vi "Camera_Config_Global_Attributes.vi"(7 "Camera":T1, 8 "error in (no error)":errorcluster, 10 "Refnum in":T3, 11 "input cluster":T2={"Pinch-valve"="", "XLP 6000 Pump"="", "Camera1"="", "Camera2"="", "Img_Capt"=FALSE, "Actuator"=FALSE, "Pump"=FALSE, "Cam 1"=FALSE, "Cam 2"=FALSE, "Empty_Refill"=FALSE, "Crop"=FALSE, "Light intensity"=0, "Exposure Time"=0.0, "Sample Name"="", "Operator"="", "Calibration 1"=path "", "Calibration 2"=path "", "Framerate"=0, "Timeout Sample"=0, "Collection date"="", "Sample size threshold"=0, "Empty start"=0, "Command"="", "Station"="", "Species Name"="", "Other Notes"="", "Aperture"=enum."Item 0", "Image Process Queue Size"=0, "Image Save Queue Size"=0, "Overload threshold"=0, "Max Framerate"=0, "Rectangle 1"={"Left"=0, "Top"=0, "Right"=0, "Bottom"=0, "Rotation"=0.0}, "Rectangle 2"={"Left"=0, "Top"=0, "Right"=0, "Bottom"=0, "Rotation"=0.0}, "Detection Region %"=200.0, "Detect 1"=path "", "Detect 2"=path "", "Max large object threshold"=500, "Open(T)/Close(F)"=FALSE, "Img_Capt Begin"=FALSE, "Dispense Speed"=0, "Flush Size"=0, "Location"="", "Latitude"="", "Longitude"="", "Determiner"="", "Sex"="", "Camera1_Img"=refnum, "Camera2_Img"=refnum, "Img1_Orig_Disp"=refnum, "Img2_Orig_Disp"=refnum, "Img1_Orig_RGB"=refnum, "Img2_Orig_RGB"=refnum, "Blue_Plane_Extract"=refnum, "Subtracted_Plane"=refnum, "Img1_Binary"=refnum, "Img2_Binary"=refnum, "Crop_Mask"=refnum, "Img1_Save"=refnum, "Img2_Save"=refnum, "Img1_Cali_Full"=refnum, "Img2_Cali_Full"=refnum, "Img1_Cali_Detect"=refnum, "Img2_Cali_Detect"=refnum, "Cam 1 queue"=refnum, "Cam 2 queue"=refnum, "Cam 1 - save queue"=refnum, "Cam 2 - save queue"=refnum, "Overlay_Ring"=0, "SystemVersion"=0, "System Serial"="", "Legacy Cam Attributes"=FALSE, "Camera Orientation 1"="", "Camera Orientation 2"="", "Pixel to mm 1"=0.0, "Pixel to mm 2"=0.0, "CAM1 Model"=enum."a2A5328-15ucBAS", "CAM2 Model"=enum."a2A5328-15ucBAS", "Flush Insect"=FALSE, "Pump Size"=FALSE, "Barcode"="", "Phase3"=FALSE, "Mega F3"="", "Container nr."=0.0, "Flush Error"=TRUE, "Start System"=FALSE, "Size Interval"=0.0, "Mun. of containers"=0.0, "Sorting sys."=FALSE, "Initial size"=0.0} {"SystemVersion" items=["Standard", "XL"]; "Overlay_Ring" items=["Session Data", "Extended Setup", "Buffer", "Camera", "Dispenser", "Stats", "Connections"]; "Flush Size" min=1; "Dispense Speed" min=1; "Rectangle 2"."Rotation" format="%.2f"; "Rectangle 2"."Left" scale=0.0..1024.0; "Rectangle 2"."Right" scale=0.0..1024.0; "Rectangle 1"."Rotation" format="%.2f"; "Rectangle 1"."Left" scale=0.0..1024.0; "Rectangle 1"."Right" scale=0.0..1024.0; "Max Framerate" min=1; "Overload threshold" min=1; "Image Save Queue Size" min=1; "Image Process Queue Size" min=1; "Empty start" min=1; "Sample size threshold" min=1; "Framerate" min=1; "Light intensity" scale=0.0..100.0}) -> (0 "error out":errorcluster, 2 "Refnum out":T3, 3 "input cluster out":T2={"Pinch-valve"="", "XLP 6000 Pump"="", "Camera1"="", "Camera2"="", "Img_Capt"=FALSE, "Actuator"=FALSE, "Pump"=FALSE, "Cam 1"=FALSE, "Cam 2"=FALSE, "Empty_Refill"=FALSE, "Crop"=FALSE, "Light intensity"=0, "Exposure Time"=0.0, "Sample Name"="", "Operator"="", "Calibration 1"=path "", "Calibration 2"=path "", "Framerate"=0, "Timeout Sample"=0, "Collection date"="", "Sample size threshold"=0, "Empty start"=0, "Command"="", "Station"="", "Species Name"="", "Other Notes"="", "Aperture"=enum."Item 0", "Image Process Queue Size"=0, "Image Save Queue Size"=0, "Overload threshold"=0, "Max Framerate"=0, "Rectangle 1"={"Left"=0, "Top"=0, "Right"=0, "Bottom"=0, "Rotation"=0.0}, "Rectangle 2"={"Left"=0, "Top"=0, "Right"=0, "Bottom"=0, "Rotation"=0.0}, "Detection Region %"=200.0, "Detect 1"=path "", "Detect 2"=path "", "Max large object threshold"=500, "Open(T)/Close(F)"=FALSE, "Img_Capt Begin"=FALSE, "Dispense Speed"=0, "Flush Size"=0, "Location"="", "Latitude"="", "Longitude"="", "Determiner"="", "Sex"="", "Camera1_Img"=refnum, "Camera2_Img"=refnum, "Img1_Orig_Disp"=refnum, "Img2_Orig_Disp"=refnum, "Img1_Orig_RGB"=refnum, "Img2_Orig_RGB"=refnum, "Blue_Plane_Extract"=refnum, "Subtracted_Plane"=refnum, "Img1_Binary"=refnum, "Img2_Binary"=refnum, "Crop_Mask"=refnum, "Img1_Save"=refnum, "Img2_Save"=refnum, "Img1_Cali_Full"=refnum, "Img2_Cali_Full"=refnum, "Img1_Cali_Detect"=refnum, "Img2_Cali_Detect"=refnum, "Cam 1 queue"=refnum, "Cam 2 queue"=refnum, "Cam 1 - save queue"=refnum, "Cam 2 - save queue"=refnum, "Overlay_Ring"=0, "SystemVersion"=0, "System Serial"="", "Legacy Cam Attributes"=FALSE, "Camera Orientation 1"="", "Camera Orientation 2"="", "Pixel to mm 1"=0.0, "Pixel to mm 2"=0.0, "CAM1 Model"=enum."a2A5328-15ucBAS", "CAM2 Model"=enum."a2A5328-15ucBAS", "Flush Insect"=FALSE, "Pump Size"=FALSE, "Barcode"="", "Phase3"=FALSE, "Mega F3"="", "Container nr."=0.0, "Flush Error"=TRUE, "Start System"=FALSE, "Size Interval"=0.0, "Mun. of containers"=0.0, "Sorting sys."=FALSE, "Initial size"=0.0} {"SystemVersion" items=["Standard", "XL"]; "Overlay_Ring" items=["Session Data", "Extended Setup", "Buffer", "Camera", "Dispenser", "Stats", "Connections"]; "Flush Size" min=1; "Dispense Speed" min=1; "Rectangle 2"."Rotation" format="%.2f"; "Rectangle 2"."Left" scale=0.0..1024.0; "Rectangle 2"."Right" scale=0.0..1024.0; "Rectangle 1"."Rotation" format="%.2f"; "Rectangle 1"."Left" scale=0.0..1024.0; "Rectangle 1"."Right" scale=0.0..1024.0; "Max Framerate" min=1; "Overload threshold" min=1; "Image Save Queue Size" min=1; "Image Process Queue Size" min=1; "Empty start" min=1; "Sample size threshold" min=1; "Framerate" min=1; "Light intensity" scale=0.0..100.0})   [LabVIEW 2024]
uses:
  controls/Data.ctl
  <vilib>/userDefined/High Color/IMAQdx.ctl
  <vilib>/vision/Image Controls.llb/IMAQ Image.ctl
  Camera_ID.ctl
  <resource>/objmgr/imaqdx.rc
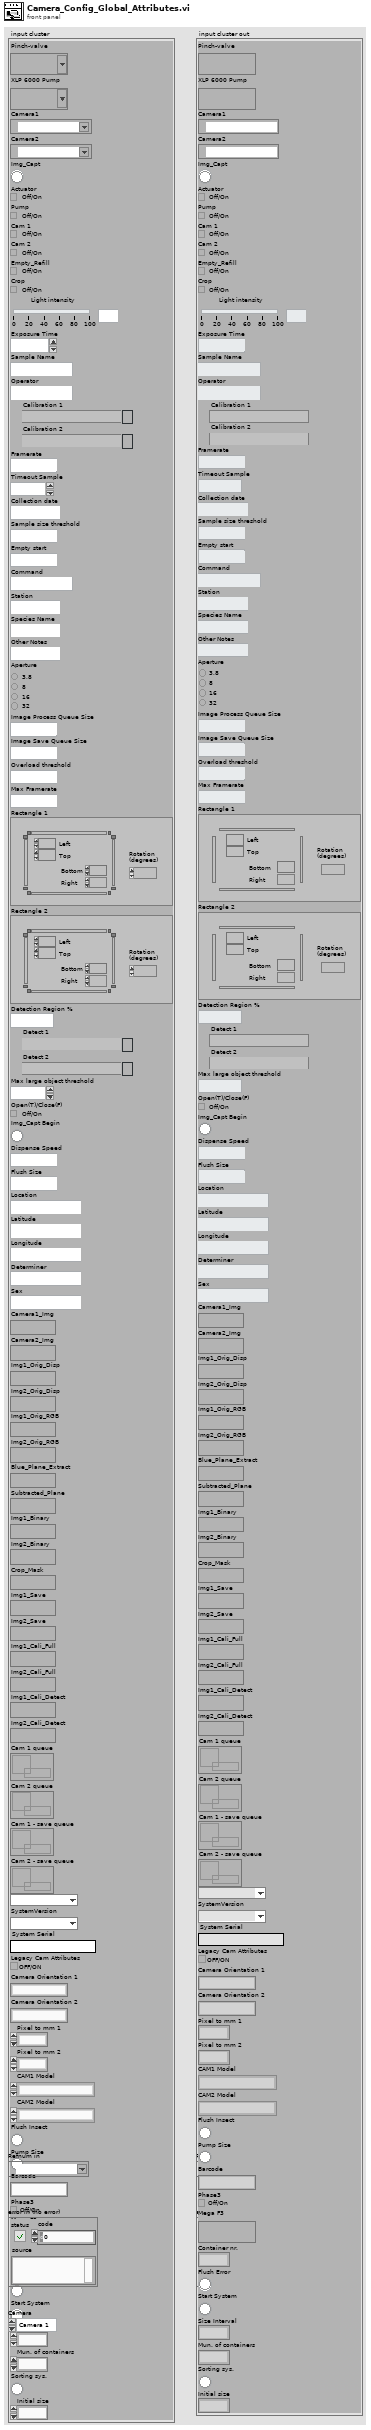
[diagram p1: front panel]
types:
  T1 = typedef "Camera_ID.ctl" = enum16{"Camera 1", "Camera 2"}
  T2 = typedef "Data.ctl" = cluster{"Pinch-valve":refnum<visa-resource-name>, "XLP 6000 Pump":refnum<visa-resource-name>, "Camera1":T3, "Camera2":T3, "Img_Capt":bool, "Actuator":bool, "Pump":bool, "Cam 1":bool, "Cam 2":bool, "Empty_Refill":bool, "Crop":bool, "Light intensity":i32, "Exposure Time":dbl, "Sample Name":string, "Operator":string, "Calibration 1":path, "Calibration 2":path, "Framerate":i32, "Timeout Sample":i32, "Collection date":string, "Sample size threshold":i32, "Empty start":u32, "Command":string, "Station":string, "Species Name":string, "Other Notes":string, "Aperture":enum32{"Item 0", "Item 1", "Item 2", "Item 3"}, "Image Process Queue Size":i32, "Image Save Queue Size":i32, "Overload threshold":i32, "Max Framerate":i32, "Rectangle 1":T4, "Rectangle 2":T4, "Detection Region %":dbl, "Detect 1":path, "Detect 2":path, "Max large object threshold":i32, "Open(T)/Close(F)":bool, "Img_Capt Begin":bool, "Dispense Speed":i32, "Flush Size":i32, "Location":string, "Latitude":string, "Longitude":string, "Determiner":string, "Sex":string, "Camera1_Img":T5, "Camera2_Img":T5, "Img1_Orig_Disp":T5, "Img2_Orig_Disp":T5, "Img1_Orig_RGB":T5, "Img2_Orig_RGB":T5, "Blue_Plane_Extract":T5, "Subtracted_Plane":T5, "Img1_Binary":T5, "Img2_Binary":T5, "Crop_Mask":T5, "Img1_Save":T5, "Img2_Save":T5, "Img1_Cali_Full":T5, "Img2_Cali_Full":T5, "Img1_Cali_Detect":T5, "Img2_Cali_Detect":T5, "Cam 1 queue":refnum<queue>, "Cam 2 queue":refnum<queue>, "Cam 1 - save queue":refnum<queue>, "Cam 2 - save queue":refnum<queue>, "Overlay_Ring":u16, "SystemVersion":u16, "System Serial":string, "Legacy Cam Attributes":bool, "Camera Orientation 1":string, "Camera Orientation 2":string, "Pixel to mm 1":dbl, "Pixel to mm 2":dbl, "CAM1 Model":enum16{"a2A5328-15ucBAS", "acA1920-155uc"}, "CAM2 Model":enum16{"a2A5328-15ucBAS", "acA1920-155uc"}, "Flush Insect":bool, "Pump Size":bool, "Barcode":string, "Phase3":bool, "Mega F3":refnum<visa-resource-name>, "Container nr.":dbl, "Flush Error":bool, "Start System":bool, "Size Interval":dbl, "Mun. of containers":dbl, "Sorting sys.":bool, "Initial size":dbl}
  T3 = typedef "IMAQdx.ctl" = refnum<k21>
  T4 = typedef "IMAQ Rectangle" = cluster{"Left":i32, "Top":i32, "Right":i32, "Bottom":i32, "Rotation":dbl}
  T5 = typedef "IMAQ Image.ctl" = refnum<image>
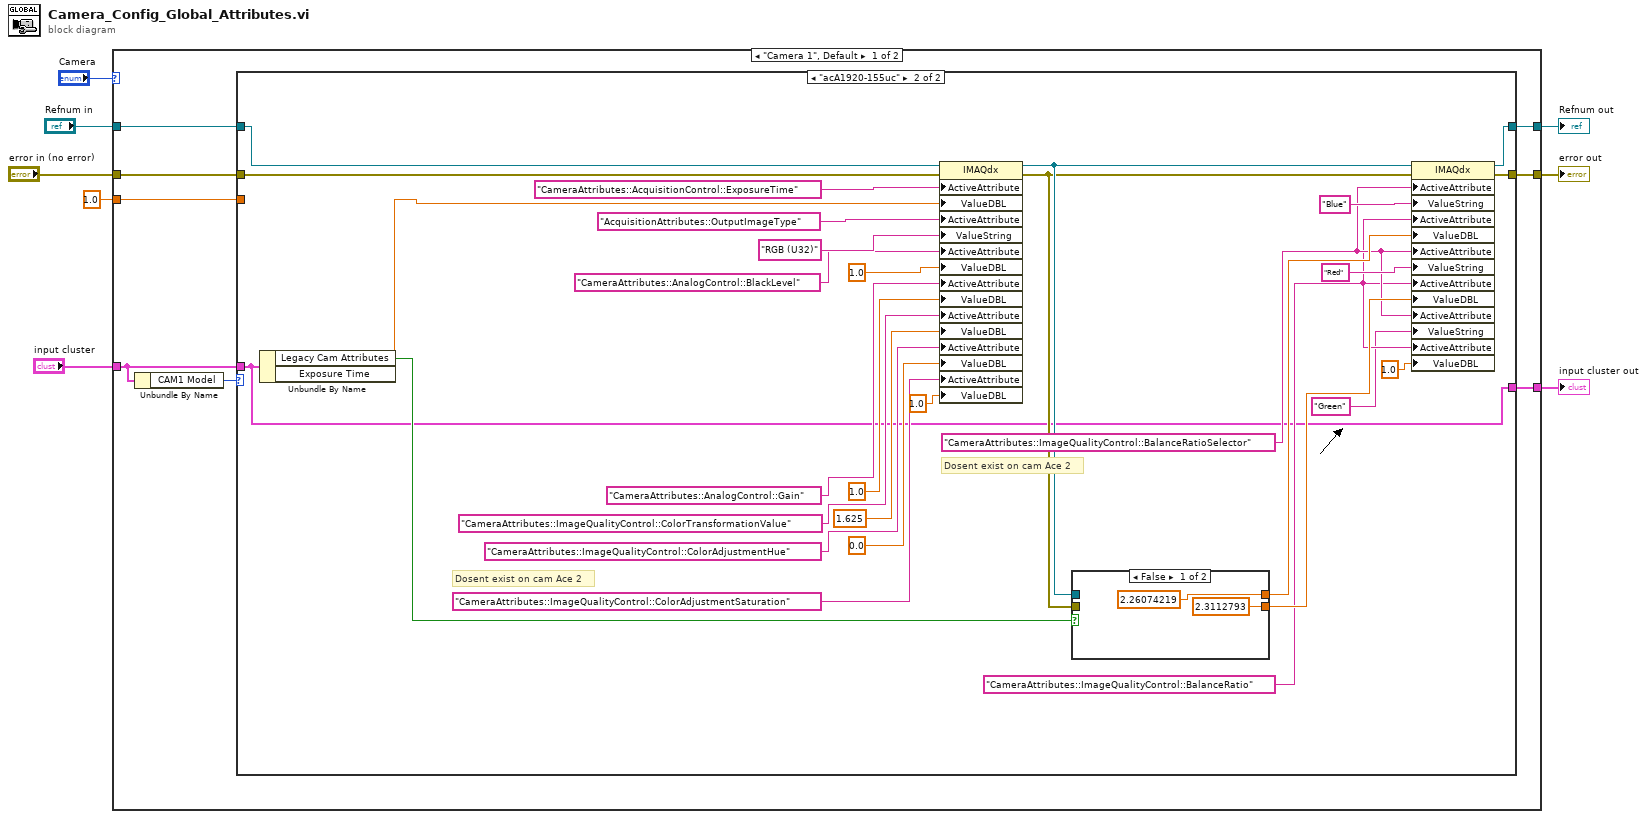
[diagram p0: block diagram]
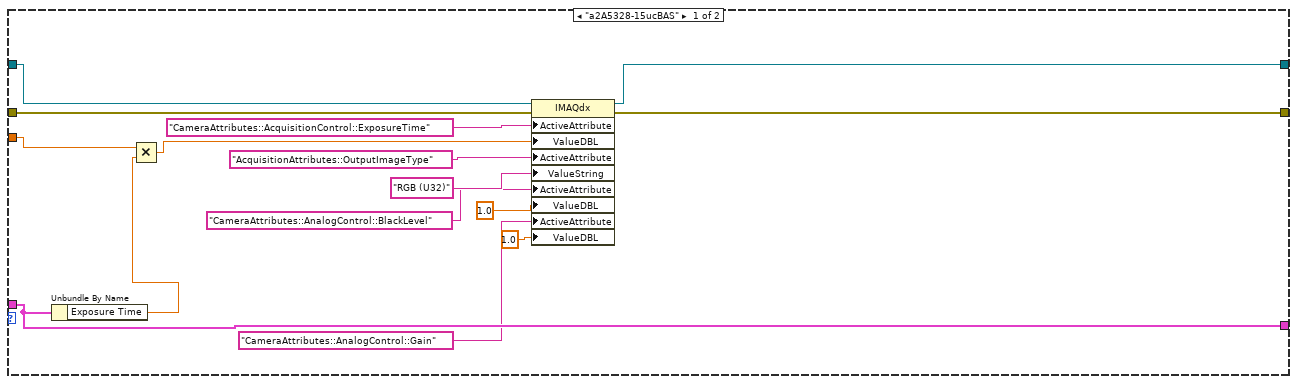
[diagram p2: hidden frame]
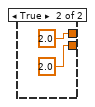
[diagram p3: hidden frame]
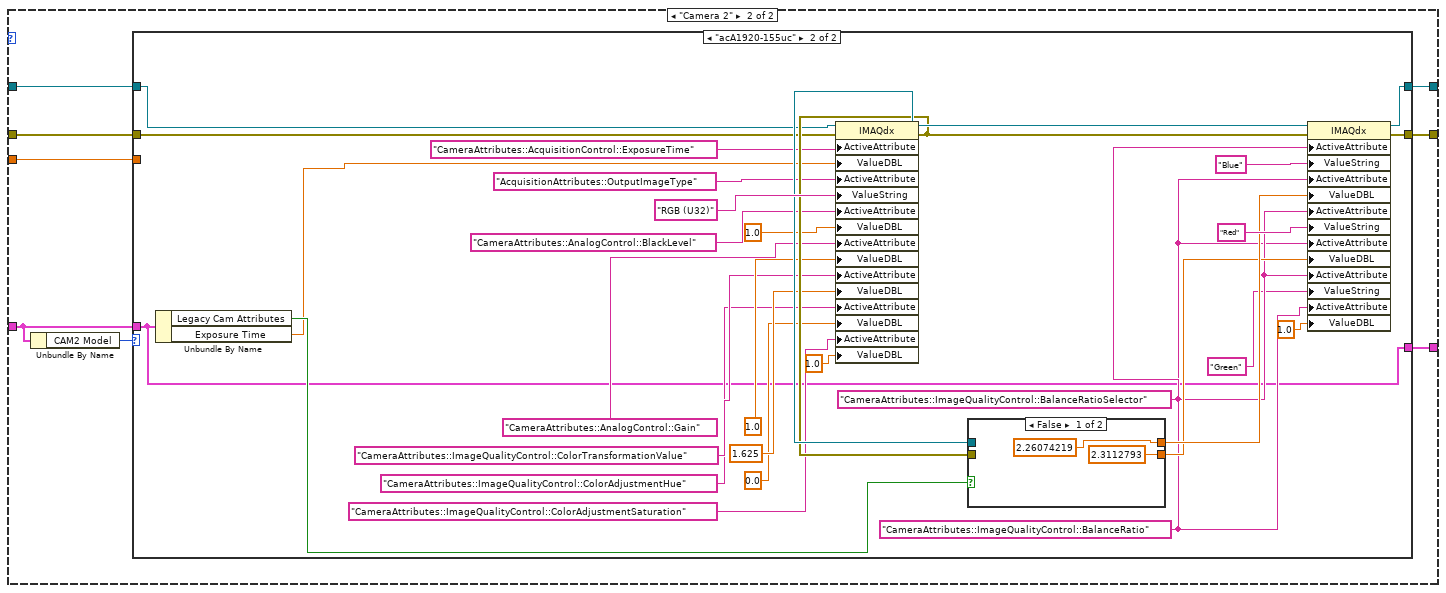
[diagram p4: hidden frame]
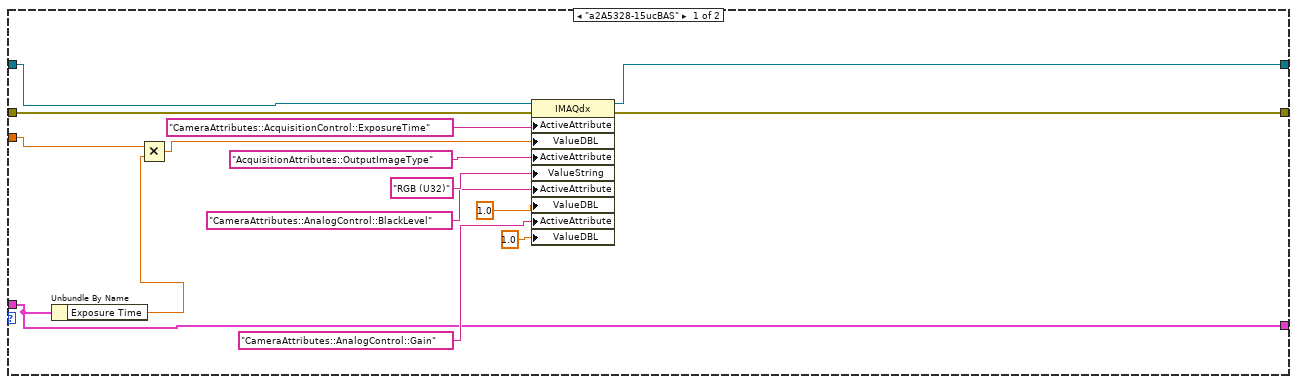
[diagram p5: hidden frame]
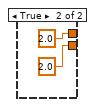
[diagram p6: hidden frame]
diagram:
  n1 = case shown="\"Camera 1\", Default" "Camera" {
    tunnel: "input cluster" -> [w13 w73]
    tunnel: "error in (no error)" -> [w14 w72]
    tunnel: [w15 w71] -> w6
    tunnel: "Refnum in" -> [w10 w69]
    tunnel: [w12 w68] -> w3
    tunnel: [w11 w67] -> w2
    tunnel: 1.0 ("x") -> [w9 w66]
    frame "Camera 1", Default {
      n2 = Unbundle By Name(w13) -> ("CAM1 Model"=w16:enum16{"a2A5328-15ucBAS", "acA1920-155uc"})
      n3 = case shown="\"acA1920-155uc\"" w16 {
        tunnel: w13 -> [w27 w34]
        tunnel: w14 -> [w31 w37]
        tunnel: [w29 w36] -> w15
        tunnel: [w27 w34] -> w12
        tunnel: [w28 w35] -> w11
        tunnel: w10 -> [w30 w33]
        tunnel: w9 -> [w19 _]
        frame "a2A5328-15ucBAS" {
          n4 = Unbundle By Name(w27) -> ("Exposure Time"=w18:dbl)
          n5 = Multiply(x=w19, y=w18) -> (x*y=w17:dbl)
          n6 = property class="IMAQdx"(reference=w30, error in=w31, "ActiveAttribute"="CameraAttributes::AcquisitionControl::ExposureTime", "ValueDBL"=w17, "ActiveAttribute"="AcquisitionAttributes::OutputImageType", "ValueString"="RGB (U32)", "ActiveAttribute"="CameraAttributes::AnalogControl::BlackLevel", "ValueDBL"=1.0, "ActiveAttribute"="CameraAttributes::AnalogControl::Gain", "ValueDBL"=1.0) -> (reference out=w28:T3, error out=w29:errorcluster)
        }
        frame "acA1920-155uc" {
          w42 = "CameraAttributes::ImageQualityControl::BalanceRatio" ("ActiveAttribute")
          w43 = "CameraAttributes::ImageQualityControl::BalanceRatioSelector" ("ActiveAttribute")
          # "Dosent exist on cam Ace 2"
          # "Dosent exist on cam Ace 2"
          n7 = Unbundle By Name(w34) -> ("Legacy Cam Attributes"=w58:bool, "Exposure Time"=w32:dbl)
          n8 = property class="IMAQdx"(reference=w33, error in=w37, "ActiveAttribute"="CameraAttributes::AcquisitionControl::ExposureTime", "ValueDBL"=w32, "ActiveAttribute"="AcquisitionAttributes::OutputImageType", "ValueString"="RGB (U32)", "ActiveAttribute"="CameraAttributes::AnalogControl::BlackLevel", "ValueDBL"=1.0, "ActiveAttribute"="CameraAttributes::AnalogControl::Gain", "ValueDBL"=1.0, "ActiveAttribute"="CameraAttributes::ImageQualityControl::ColorTransformationValue", "ValueDBL"=1.625, "ActiveAttribute"="CameraAttributes::ImageQualityControl::ColorAdjustmentHue", "ValueDBL"=0.0, "ActiveAttribute"="CameraAttributes::ImageQualityControl::ColorAdjustmentSaturation", "ValueDBL"=1.0) -> (reference out=w60:T3, error out=w59:errorcluster)
          n9 = case shown="False" w58 {
            tunnel: w60 -> [_ _]
            tunnel: w59 -> [_ _]
            tunnel: [2.26074219 ("ValueDBL") 2.0 ("ValueDBL")] -> w55
            tunnel: [2.3112793 ("ValueDBL") 2.0 ("ValueDBL")] -> w54
            frame False {
            }
            frame True {
            }
          }
          n10 = property class="IMAQdx"(reference=w60, error in=w59, "ActiveAttribute"=w43, "ValueString"="Blue", "ActiveAttribute"=w42, "ValueDBL"=w55, "ActiveAttribute"=w43, "ValueString"="Red", "ActiveAttribute"=w42, "ValueDBL"=w54, "ActiveAttribute"=w43, "ValueString"="Green", "ActiveAttribute"=w42, "ValueDBL"=1.0) -> (reference out=w35:T3, error out=w36:errorcluster)
        }
      }
    }
    frame "Camera 2" {
      n11 = Unbundle By Name(w73) -> ("CAM2 Model"=w70:enum16{"a2A5328-15ucBAS", "acA1920-155uc"})
      n12 = case shown="\"acA1920-155uc\"" w70 {
        tunnel: w73 -> [w79 w90]
        tunnel: w72 -> [w81 w94]
        tunnel: [w78 w93] -> w71
        tunnel: w69 -> [w80 w91]
        tunnel: [w79 w90] -> w68
        tunnel: [w77 w92] -> w67
        tunnel: w66 -> [w74 _]
        frame "a2A5328-15ucBAS" {
          n13 = Unbundle By Name(w79) -> ("Exposure Time"=w76:dbl)
          n14 = Multiply(x=w74, y=w76) -> (x*y=w75:dbl)
          n15 = property class="IMAQdx"(reference=w80, error in=w81, "ActiveAttribute"="CameraAttributes::AcquisitionControl::ExposureTime", "ValueDBL"=w75, "ActiveAttribute"="AcquisitionAttributes::OutputImageType", "ValueString"="RGB (U32)", "ActiveAttribute"="CameraAttributes::AnalogControl::BlackLevel", "ValueDBL"=1.0, "ActiveAttribute"="CameraAttributes::AnalogControl::Gain", "ValueDBL"=1.0) -> (reference out=w77:T3, error out=w78:errorcluster)
        }
        frame "acA1920-155uc" {
          w99 = "CameraAttributes::ImageQualityControl::BalanceRatio" ("ActiveAttribute")
          w100 = "CameraAttributes::ImageQualityControl::BalanceRatioSelector" ("ActiveAttribute")
          n16 = Unbundle By Name(w90) -> ("Legacy Cam Attributes"=w115:bool, "Exposure Time"=w89:dbl)
          n17 = property class="IMAQdx"(reference=w91, error in=w94, "ActiveAttribute"="CameraAttributes::AcquisitionControl::ExposureTime", "ValueDBL"=w89, "ActiveAttribute"="AcquisitionAttributes::OutputImageType", "ValueString"="RGB (U32)", "ActiveAttribute"="CameraAttributes::AnalogControl::BlackLevel", "ValueDBL"=1.0, "ActiveAttribute"="CameraAttributes::AnalogControl::Gain", "ValueDBL"=1.0, "ActiveAttribute"="CameraAttributes::ImageQualityControl::ColorTransformationValue", "ValueDBL"=1.625, "ActiveAttribute"="CameraAttributes::ImageQualityControl::ColorAdjustmentHue", "ValueDBL"=0.0, "ActiveAttribute"="CameraAttributes::ImageQualityControl::ColorAdjustmentSaturation", "ValueDBL"=1.0) -> (reference out=w117:T3, error out=w116:errorcluster)
          n18 = case shown="False" w115 {
            tunnel: w117 -> [_ _]
            tunnel: w116 -> [_ _]
            tunnel: [2.26074219 ("ValueDBL") 2.0 ("ValueDBL")] -> w112
            tunnel: [2.3112793 ("ValueDBL") 2.0 ("ValueDBL")] -> w111
            frame False {
            }
            frame True {
            }
          }
          n19 = property class="IMAQdx"(reference=w117, error in=w116, "ActiveAttribute"=w100, "ValueString"="Blue", "ActiveAttribute"=w99, "ValueDBL"=w112, "ActiveAttribute"=w100, "ValueString"="Red", "ActiveAttribute"=w99, "ValueDBL"=w111, "ActiveAttribute"=w100, "ValueString"="Green", "ActiveAttribute"=w99, "ValueDBL"=1.0) -> (reference out=w92:T3, error out=w93:errorcluster)
        }
      }
    }
  }
  "error out" <- w6
  "input cluster out" <- w3
  "Refnum out" <- w2
